vi "Aim_At_Target.vi"() -> ()   [LabVIEW 2019]
uses:
  <vilib>/Rock Robotics/WPI/Joystick/XBox Buttons Indexer.ctl
  <vilib>/Rock Robotics/WPI/Joystick/XBox Axes Indexer.ctl
  <vilib>/Rock Robotics/WPI/ThirdParty/JAS_Junk/TrajLib/PIDController_AtSetpoint.vi
  <vilib>/Rock Robotics/WPI/ThirdParty/JAS_Junk/TrajLib/PIDController_SetPIDF.vi
  <vilib>/Rock Robotics/WPI/ThirdParty/JAS_Junk/TrajLib/PIDController_SetDerivativeFilter.vi
  <vilib>/Rock Robotics/WPI/ThirdParty/JAS_Junk/TrajLib/PIDController_SetIntegratorRange.vi
  <vilib>/Rock Robotics/WPI/ThirdParty/JAS_Junk/TrajLib/PIDController_SetTolerancePandV.vi
  <vilib>/Rock Robotics/WPI/ThirdParty/JAS_Junk/TrajLib/PIDController_DisableContinousInput.vi
  <vilib>/Rock Robotics/WPI/ThirdParty/JAS_Junk/TrajLib/PIDController_EnableContinousInput.vi
  <vilib>/Rock Robotics/WPI/ThirdParty/JAS_Junk/TrajLib/PIDController_Reset.vi
  <vilib>/Rock Robotics/WPI/ThirdParty/JAS_Junk/TrajLib/PIDController_New.vi
  <vilib>/Rock Robotics/WPI/ThirdParty/JAS_Junk/TrajLib/PIDController_SetOutputLimits.vi
  <vilib>/Rock Robotics/WPI/ThirdParty/JAS_Junk/TrajLib/ControllerUtil_GetModulusError.vi
  <vilib>/Rock Robotics/WPI/ThirdParty/JAS_Junk/TrajLib/PIDController_NewPeriod.vi
  <vilib>/Rock Robotics/SystemInterfaces/NetworkCommunication/NetComm_UsageReport_report.vi
  <vilib>/Rock Robotics/WPI/Utilities/WPI_GetSetVariantRefNum.vi
  <vilib>/Rock Robotics/Network Tables/NT Write Boolean.vi
  <vilib>/Rock Robotics/WPI/Joystick/WPI_JoystickArcadeMapping.vi
  <vilib>/Rock Robotics/Network Tables/NT Write Number.vi
  <vilib>/Rock Robotics/WPI/ThirdParty/JAS_Junk/TrajLib/Util_LibraryGlobals.vi
  <vilib>/Rock Robotics/WPI/ThirdParty/JAS_Junk/TrajLib/PIDController_AdvCalculate_FF_Sp_Pv.vi
  <vilib>/Rock Robotics/Network Tables/NT Write Numeric Array.vi
  <vilib>/Rock Robotics/WPI/ThirdParty/PhotonVisionLib/PhotonVisionLib.lvlib
  <vilib>/Rock Robotics/WPI/ThirdParty/JAS_Junk/TrajLib/Trajectory_Library.lvlib
panel:
  out "Auto Aim\nSelected":bool
  out "TargetFound":bool
  out "Yaw":dbl
  out "DistanceToTarget Meters":dbl
  out "Right Motor Demand":dbl format="%14.4f"
  out "Left Motor Demand":dbl format="%14.4f"
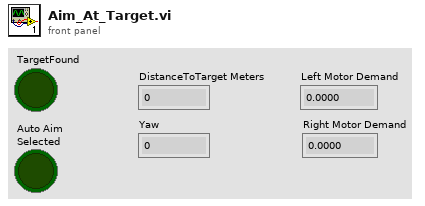
[diagram p1: front panel]
types:
  T1 = typedef "WPI_RobotDriveDevRef.ctl" = cluster{"DevStatus":errorcluster, "Motors[]":T2[], "Square Inputs":bool, "Max Output":dbl}
  T2 = typedef "WPI_MotorControlDeviceRef.ctl" = cluster{"DeviceStatus":errorcluster, "Type":T3, "PWM":cluster{"PWM Channel":T4, "DeadBand":T5}, "CAN":cluster{"Device Number":u8, "SetOutput VI Ref":variant, "GetOutput VI Ref":variant, "Enable VI Ref":variant, "Disable VI Ref":variant, "Data":variant}, "Invert":bool, "DIO PWM":cluster{"PWM \"Enable\" Channel":T4, "DIOChannel":T6, "PWM Rate":dbl}}
  T3 = typedef "WPI_MotorControlType.ctl" = enum16{"PWM", "CAN", "DIO PWM"}
  T4 = typedef "FPGA_DIOPWMChannel.ctl" = enum8{"PWM 0", "PWM 1", "PWM 2", "PWM 3", "PWM 4", "PWM 5", "PWM 6", "PWM 7", "PWM 8", "PWM 9", "PWM MXP 0", "PWM MXP 1", "PWM MXP 2", "PWM MXP 3", "PWM MXP 4", "PWM MXP 5", "PWM MXP 6", "PWM MXP 7", "PWM MXP 8", "PWM MXP 9", "Invalid"}
  T5 = typedef "WPI_PWMDeadband.ctl" = cluster{"Name":string, "maxPositivePwm":i32, "minPositivePwm":i32, "centerPwm":i32, "maxNegativePwm":i32, "minNegativePwm":i32, "angularRange":u16}
  T6 = typedef "FPGA_DIOChannel.ctl" = enum8{"DIO 0", "DIO 1", "DIO 2", "DIO 3", "DIO 4", "DIO 5", "DIO 6", "DIO 7", "DIO 8", "DIO 9", "DIO MXP 0", "DIO MXP 1", "DIO MXP 2", "DIO MXP 3", "DIO MXP 4", "DIO MXP 5", "DIO MXP 6", "DIO MXP 7", "DIO MXP 8", "DIO MXP 9", "DIO MXP 10", "DIO MXP 11", "DIO MXP 12", "DIO MXP 13", "DIO MXP 14", "DIO MXP 15", "SPI Port CS1", "SPI Port CS2", "SPI Port CS3", "SPI Port MISO", "SPI Port MOSI", "Invalid"}
  T7 = typedef "WPI_JoystickDevRef.ctl" = cluster{"Device":T8}
  T8 = typedef "WPI_JoystickDeviceEnum.ctl" = enum16{"USB 0", "USB 1", "USB 2", "USB 3", "USB 4", "USB 5"}
  T9 = typedef "XBox Axes Indexer.ctl" = enum16{"Left X", "Left Y", "Left Trigger", "Right Trigger", "Right X", "Right Y"}
  T10 = typedef "XBox Buttons Indexer.ctl" = enum16{"A", "B", "X", "Y", "Left Bumper", "Right Bumper", "Back", "Start", "Left Joystick", "Right Joystick"}
  T11 = typedef "PhotonVisionLib.lvlib/PhotonPipelineResultType.ctl" = cluster{"TargetCount":i32, "Latency_MilliSec":dbl, "Targets":T12[]}
  T12 = typedef "PhotonVisionLib.lvlib/PhotonTrackedTargetType.ctl" = cluster{"Yaw":dbl, "Pitch":dbl, "Area":dbl, "Skew":dbl, "TargetCorners":T13[], "CameraToTarget":T14}
  T13 = typedef "PhotonVisionLib.lvlib/TargetCornerType.ctl" = cluster{"X":dbl, "Y":dbl}
  T14 = typedef "Trajectory_Library.lvlib/TRANSFORM2D.ctl" = cluster{"TRANSLATION":T15, "ROTATION":T16}
  T15 = typedef "Trajectory_Library.lvlib/TRANSLATION2D.ctl" = cluster{"X":dbl, "Y":dbl}
  T16 = typedef "Trajectory_Library.lvlib/ROTATION2D.ctl" = cluster{"VALUE":dbl, "COS":dbl, "SIN":dbl}
  T17 = typedef "Trajectory_Library.lvlib/PID_ADV_LIMITS.ctl" = cluster{"MaxInput":dbl, "MinInput":dbl, "Continuous":bool, "MaxOutput":dbl, "MinOutput":dbl}
  T18 = typedef "Trajectory_Library.lvlib/PID_ADV_TUNING.ctl" = cluster{"Kf":dbl, "Kp":dbl, "Ki":dbl, "Kd":dbl, "MaximumIntegral":dbl, "MinimumIntegral":dbl, "Filter Derivative":bool}
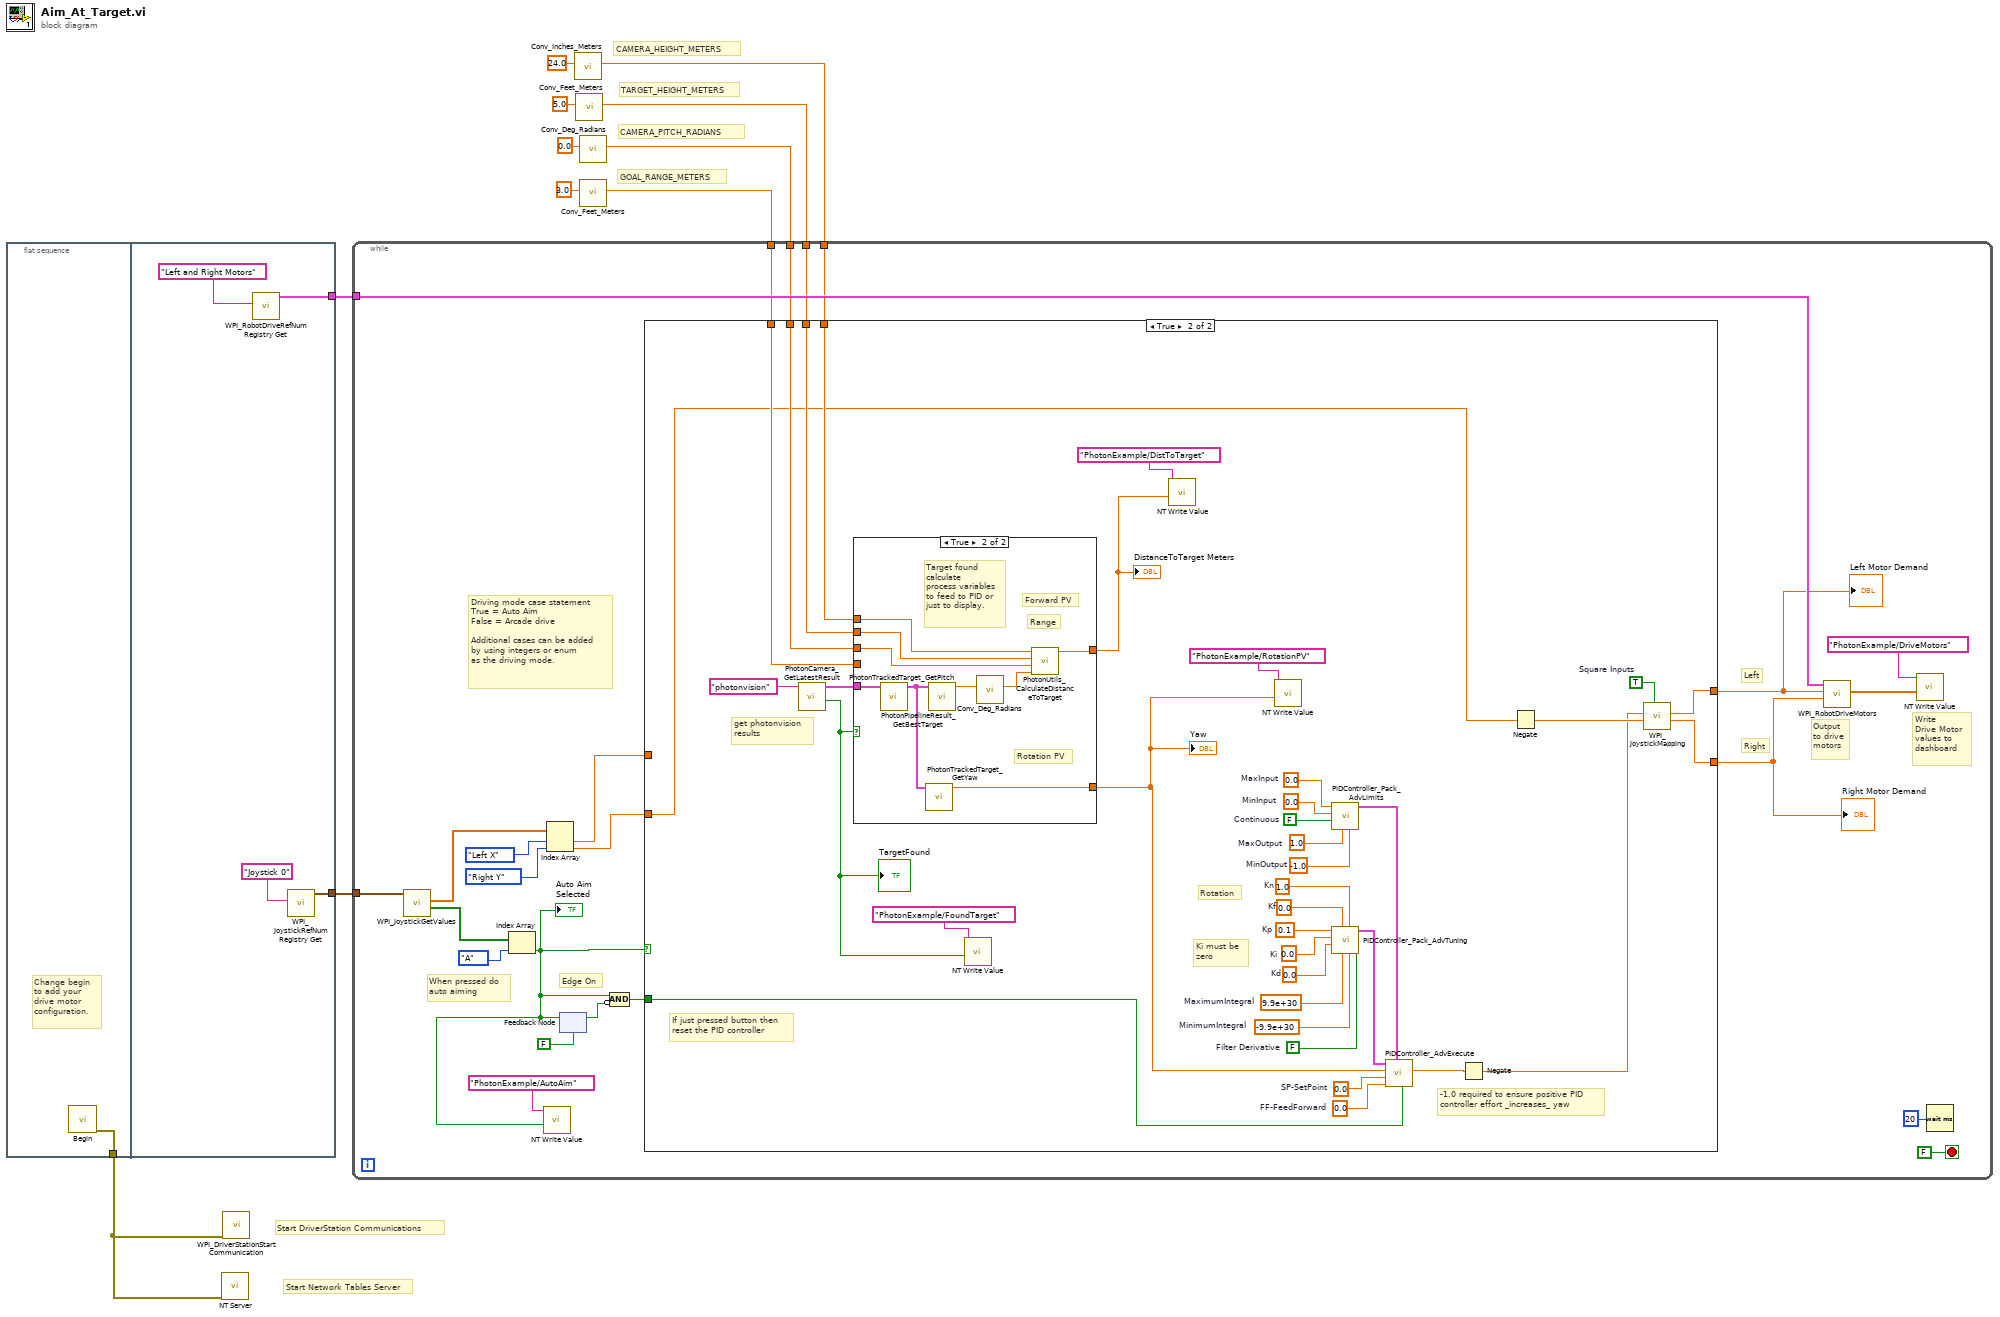
[diagram p0: block diagram]
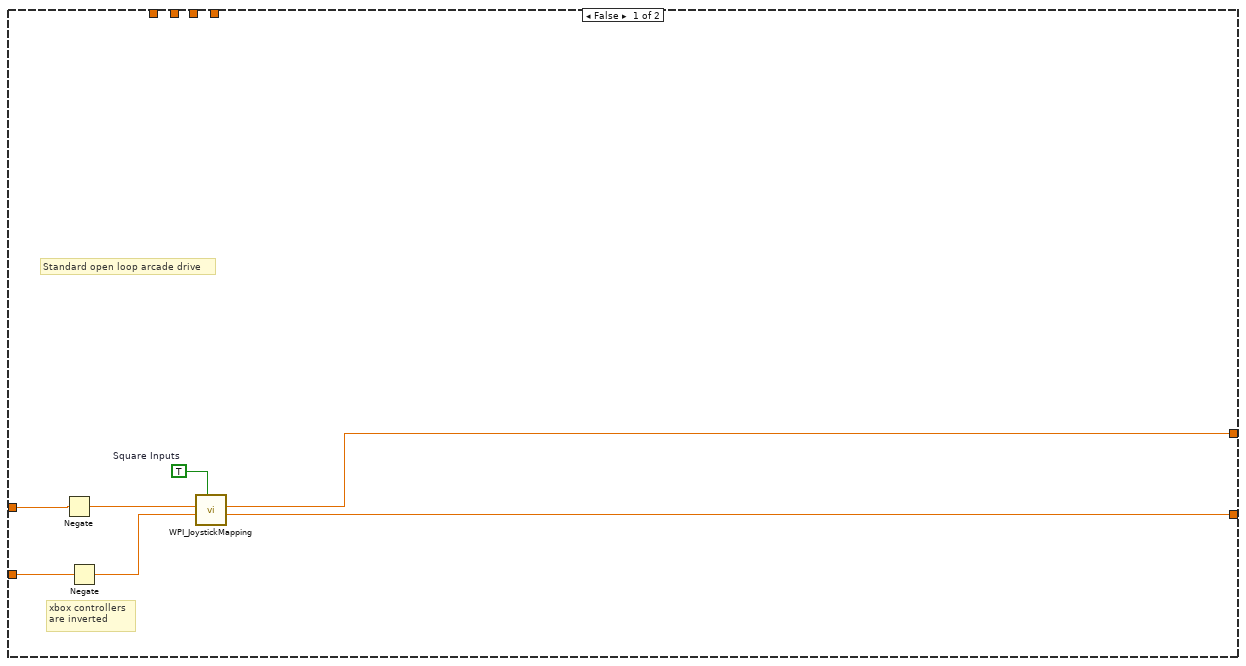
[diagram p2: hidden frame]
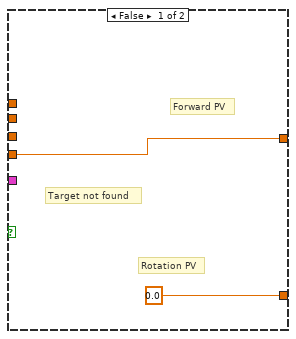
[diagram p3: hidden frame]
diagram:
  # "GOAL_RANGE_METERS"
  # "CAMERA_PITCH_RADIANS"
  # "TARGET_HEIGHT_METERS"
  # "CAMERA_HEIGHT_METERS"
  # "Start Network Tables Server"
  # "Start DriverStation Communications"
  n1 = flat-sequence {
    tunnel: [w12] -> w11
    tunnel: [w15] -> w10
    tunnel: [w13] -> w9
    frame #0 {
      # "Change begin\nto add your \ndrive motor\nconfiguration."
      n2 = call "Begin.vi"() -> ("error out"=w12:errorcluster)  [unwired: 11 in]
    }
    frame #1 {
      n3 = call <vilib>:"WPI_RobotDriveRefNum Registry Get.vi"("refnum name"="Left and Right Motors") -> ("RobotDriveDevRef"=w13:T1)  [unwired: 9 in, 1 out]
      n4 = call <vilib>:"WPI_JoystickRefNum Registry Get.vi"("refnum name"="Joystick 0") -> ("JoystickDevRef"=w15:T7)  [unwired: 9 in, 1 out]
    }
  }
  n5 = call <vilib>:"NT Server.vi"("error in (no error)"=w11) -> ()  [unwired: 11 in]
  n6 = call <vilib>:"WPI_DriverStationStart Communication.vi"("error in (no error)"=w11) -> ()  [unwired: 11 in]
  n7 = call <vilib>:"Conv_Inches_Meters.vi"("INCH"=24.0) -> ("Meters"=w4:dbl)  [unwired: 10 in]
  n8 = call <vilib>:"Conv_Feet_Meters.vi"("Feet"=5.0) -> ("Meters"=w3:dbl)  [unwired: 10 in]
  n9 = call <vilib>:"Conv_Feet_Meters.vi"("Feet"=3.0) -> ("Meters"=w1:dbl)  [unwired: 10 in]
  n10 = call <vilib>:"Conv_Deg_Radians.vi"("Degress"=0.0) -> ("Radians"=w2:dbl)  [unwired: 10 in]
  n11 = while {
    tunnel: w10 -> [w39]
    tunnel: w9 -> [w31]
    tunnel: w4 -> [w22]
    tunnel: w3 -> [w21]
    tunnel: w2 -> [w20]
    tunnel: w1 -> [w19]
    stop <- FALSE stop-if-true
    # "Write \nDrive Motor\nvalues to \ndashboard"
    # "Output\nto drive\nmotors"
    # "Edge On"
    # "Right"
    # "Left"
    # "Driving mode case statement\nTrue = Auto Aim\nFalse = Arcade drive\n\nAdditional cases can be added\nby using integers or enum\nas the driving mode."
    # "When pressed do\nauto aiming"
    n12 = call <vilib>:"WPI_JoystickGetValues.vi"("JoystickDevRef"=w39) -> ("Buttons"=w38:bool[], "Axes"=w37:dbl[])  [unwired: 6 in, 3 out]
    n13 = Index Array(array=w38, index=XBox_Buttons_Indexer."A" ("XBox Buttons")) -> (element=w17:bool)
    "Auto Aim\nSelected" <- w17
    n14 = call-poly <vilib>:"NT Write Value.vi"("Boolean"=w17, "Name"="PhotonExample/AutoAim") -> ()  [unwired: 9 in, 1 out]
    n15 = Index Array(array=w37, index #1=XBox_Axes_Indexer."Left X" ("XBox Axes"), index #2=XBox_Axes_Indexer."Right Y" ("XBox Axes")) -> (element #1=w33:dbl, element #2=w32:dbl)
    n16 = feedback-in #1(w17) -> ()
    n17 = feedback #1(FALSE) -> (w28:bool)
    n18 = Compound Arithmetic op=AND(w17, invert w28) -> (w29:bool)
    n19 = case shown="True" w17 {
      tunnel: w33 -> [w47 _]
      tunnel: w32 -> [w46 w48]
      tunnel: [w42 w82] -> w30
      tunnel: [w41 w81] -> w23
      tunnel: w29 -> [_ w63]
      tunnel: w22 -> [_ w61]
      tunnel: w21 -> [_ w60]
      tunnel: w20 -> [_ w59]
      tunnel: w19 -> [_ w58]
      frame False {
        w43 = TRUE  # Square Inputs
        # "Standard open loop arcade drive"
        # "xbox controllers\nare inverted"
        n20 = Negate(x=w47) -> (-x=w45:dbl)
        n21 = Negate(x=w46) -> (-x=w44:dbl)
        n22 = call-poly <vilib>:"WPI_JoystickMapping.vi"("Square Inputs"=w43, "Y axis value"=w44, "X axis value"=w45) -> ("Right Motor Value"=w41:dbl, "Left Motor Value"=w42:dbl)  [unwired: 7 in]
      }
      frame True {
        w62 = 0.0  # FF-FeedForward
        w64 = 0.0  # SP-SetPoint
        w80 = 1.0  # Kn
        w79 = 0.1  # Kp
        w78 = 0.0  # Ki
        w77 = 0.0  # Kd
        w76 = 0.0  # Kf
        w75 = 9.9e+30  # MaximumIntegral
        w74 = -9.9e+30  # MinimumIntegral
        w73 = FALSE  # Filter Derivative
        w71 = 0.0  # MinInput
        w70 = FALSE  # Continuous
        w69 = 1.0  # MaxOutput
        w72 = -1.0  # MinOutput
        w68 = 0.0  # MaxInput
        w83 = TRUE  # Square Inputs
        # "-1.0 required to ensure positive PID \ncontroller effort _increases_ yaw"
        # "Ki must be \nzero"
        # "If just pressed button then\nreset the PID controller"
        # "Rotation"
        # "get photonvision\nresults"
        n23 = call <vilib>:"PhotonCamera_GetLatestResult.vi"("CameraName"="photonvision") -> ("HasTargets"=w53:bool, "PipelineResult"=w65:T11)  [unwired: 9 in]
        "TargetFound" <- w53
        n24 = case shown="True" w53 {
          tunnel: w65 -> [_ w95]
          tunnel: [w85 w91] -> w49
          tunnel: [0.0 w90] -> w50
          tunnel: w61 -> [_ w87]
          tunnel: w60 -> [_ w88]
          tunnel: w59 -> [_ w89]
          tunnel: w58 -> [w85 _]
          frame False {
            # "Forward PV"
            # "Rotation PV"
            # "Target not found"
          }
          frame True {
            # "Target found\ncalculate\nprocess variables\nto feed to PID or\njust to display."
            # "Range"
            # "Forward PV"
            # "Rotation PV"
            n25 = call <vilib>:"PhotonPipelineResult_GetBestTarget.vi"("PhotonPipelineResult"=w95) -> ("PhotonTrackedTarget"=w92:T12)  [unwired: 10 in]
            n26 = call <vilib>:"PhotonTrackedTarget_GetYaw.vi"("TrackedTarget"=w92) -> ("Yaw"=w90:dbl)  [unwired: 10 in]
            n27 = call <vilib>:"PhotonTrackedTarget_GetPitch.vi"("TrackedTarget"=w92) -> ("Pitch"=w94:dbl)  [unwired: 10 in]
            n28 = call <vilib>:"Conv_Deg_Radians.vi"("Degress"=w94) -> ("Radians"=w93:dbl)  [unwired: 10 in]
            n29 = call <vilib>:"PhotonUtils_CalculateDistanceToTarget.vi"("TargetPitch_Radians"=w93, "CameraPitch_Radians"=w89, "TargetHeight_Meters"=w88, "CameraHeight_Meters"=w87) -> ("DistanceToTarget_Meters"=w91:dbl)  [unwired: 7 in]
          }
        }
        "DistanceToTarget Meters" <- w49
        "Yaw" <- w50
        n30 = call-poly <vilib>:"NT Write Value.vi"("Boolean"=w53, "Name"="PhotonExample/FoundTarget") -> ()  [unwired: 9 in, 1 out]
        n31 = call-poly <vilib>:"NT Write Value.vi"("Numeric"=w49, "Name"="PhotonExample/DistToTarget") -> ()  [unwired: 9 in, 1 out]
        n32 = call-poly <vilib>:"NT Write Value.vi"("Numeric"=w50, "Name"="PhotonExample/RotationPV") -> ()  [unwired: 9 in, 1 out]
        n33 = call <vilib>:"PIDController_Pack_AdvLimits.vi"("MinOutput"=w72, "MaxOutput"=w69, "Continuous"=w70, "MinInput"=w71, "MaxInput"=w68) -> ("Adv PID Limits"=w66:T17)  [unwired: 6 in]
        n34 = call <vilib>:"PIDController_Pack_AdvTuning.vi"("Filter Derivative"=w73, "MinimumIntegral"=w74, "Kn"=w80, "MaximumIntegral"=w75, "Kf"=w76, "Kd"=w77, "Ki"=w78, "Kp"=w79) -> ("Adv PID Tuning"=w67:T18)  [unwired: 3 in]
        n35 = call <vilib>:"PIDController_AdvExecute.vi"("Reset"=w63, "Adv PID Limits"=w66, "FF-FeedForward"=w62, "SP-SetPoint"=w64, "PV-Measurement"=w50, "Adv PID Tuning"=w67) -> ("CO-ControlOutput"=w56:dbl)  [unwired: 3 in, 2 out]
        n36 = Negate(x=w56) -> (-x=w55:dbl)
        n37 = Negate(x=w48) -> (-x=w57:dbl)
        n38 = call-poly <vilib>:"WPI_JoystickMapping.vi"("Square Inputs"=w83, "Y axis value"=w57, "X axis value"=w55) -> ("Right Motor Value"=w81:dbl, "Left Motor Value"=w82:dbl)  [unwired: 7 in]
      }
    }
    "Left Motor Demand" <- w30
    "Right Motor Demand" <- w23
    n39 = call <vilib>:"WPI_RobotDriveMotors.vi"("RightSpeed"=w23, "LeftSpeed"=w30, "RobotDriveDevRef"=w31) -> ("Motor Values"=w25:dbl[])  [unwired: 6 in, 2 out]
    n40 = call-poly <vilib>:"NT Write Value.vi"("Numeric Array"=w25, "Name"="PhotonExample/DriveMotors") -> ()  [unwired: 9 in, 1 out]
    n41 = Wait (ms)(milliseconds to wait=u32 20) -> ()  [unwired: 1 out]
  }
